vi "AdjustScale.vi"(6 "error in (no error)":errorcluster, 7 "Action":enum16{"Init", "Ignore", "Set Scale"}(ring), 8 "Input Red":dbl, 9 "Red Refnum":refnum<vi>, 10 "Input Blue":dbl, 11 "Blue Refnum":refnum<vi>) -> (4 "error out":errorcluster)   [LabVIEW 2013, in "main.lvlib"]
uses:
  main.lvlib
  <vilib>/Utility/miscctls.llb/LVRangeTypeDef.ctl
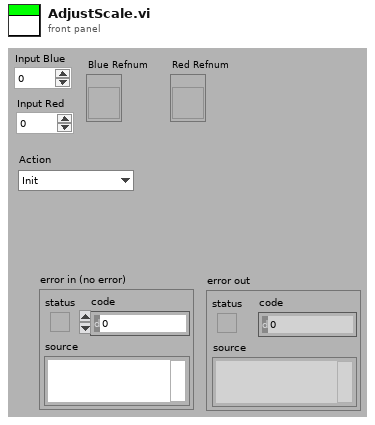
[diagram p1: front panel]
types:
  T1 = typedef "LVRangeTypeDef.ctl" = cluster{"Minimum":dbl, "Maximum":dbl, "Increment":dbl, "Minor Increment":dbl, "Start":dbl}
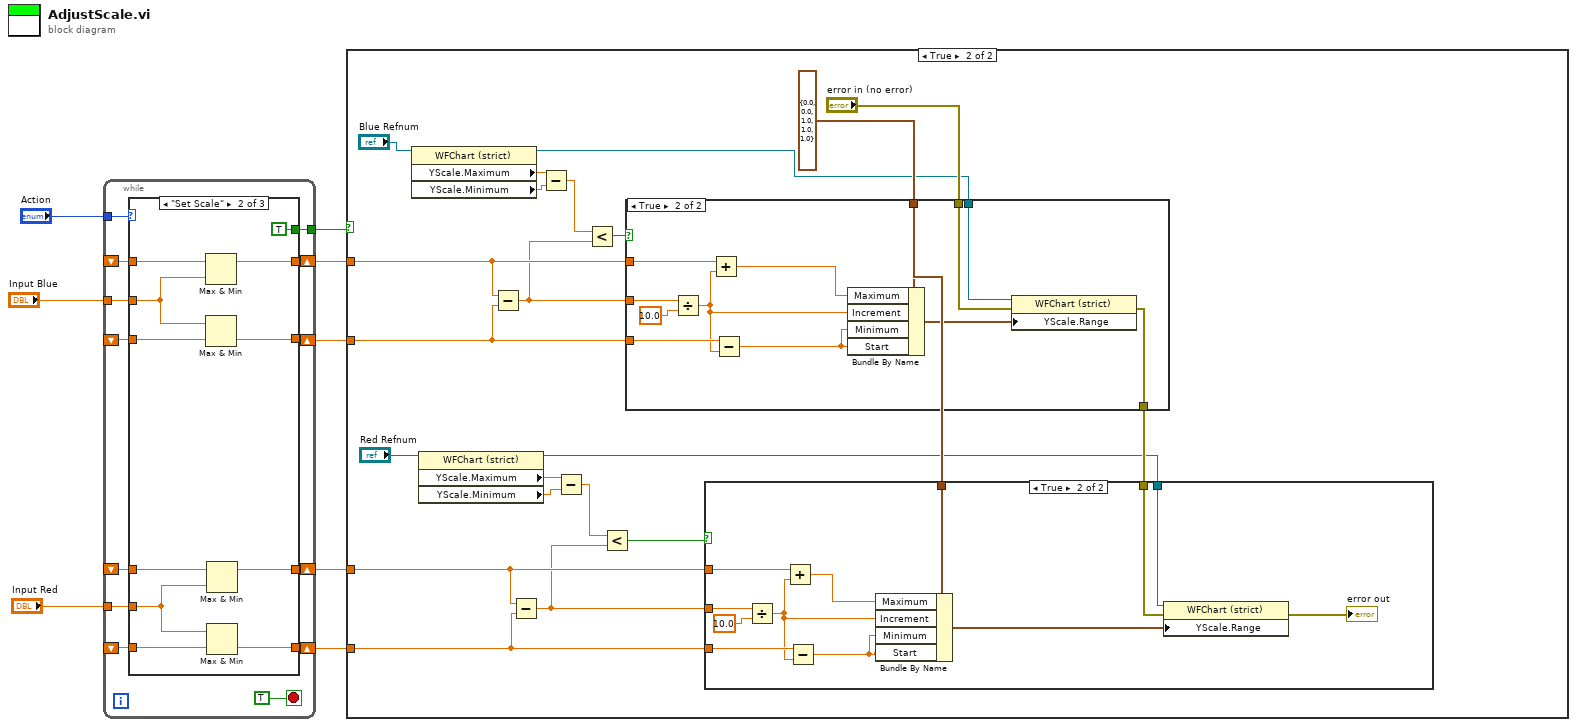
[diagram p0: block diagram]
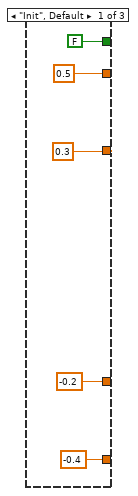
[diagram p5: hidden frame]
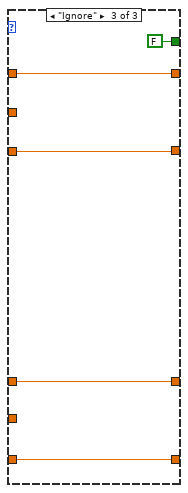
[diagram p6: hidden frame]
diagram:
  n1 = while {
    shift-right: [w19] -> w6
    shift-left: _ -> [w20]
    tunnel: "Input Blue" -> [w21]
    tunnel: "Action" -> [w17]
    shift-right: [w16] -> w5
    shift-left: _ -> [w15]
    shift-right: [w11] -> w3
    shift-left: _ -> [w13]
    shift-right: [w10] -> w2
    shift-left: _ -> [w14]
    tunnel: "Input Red" -> [w12]
    tunnel: [w9] -> w1
    stop <- TRUE stop-if-true
    n2 = case shown="\"Set Scale\"" w17 {
      tunnel: w21 -> [_ w33 _]
      tunnel: w20 -> [_ w37 w41]
      tunnel: [0.5 w36 w41] -> w19
      tunnel: [0.3 w35 w40] -> w16
      tunnel: w15 -> [_ w34 w40]
      tunnel: w14 -> [_ w32 w38]
      tunnel: w13 -> [_ w31 w39]
      tunnel: w12 -> [_ w30 _]
      tunnel: [-0.2 w29 w39] -> w11
      tunnel: [-0.4 w28 w38] -> w10
      tunnel: [FALSE TRUE FALSE] -> w9
      frame "Init", Default {
      }
      frame "Set Scale" {
        n3 = Max & Min(x=w37, y=w33) -> (max(x,y)=w36:dbl)  [unwired: 1 out]
        n4 = Max & Min(x=w33, y=w34) -> (min(x,y)=w35:dbl)  [unwired: 1 out]
        n5 = Max & Min(x=w31, y=w30) -> (max(x,y)=w29:dbl)  [unwired: 1 out]
        n6 = Max & Min(x=w30, y=w32) -> (min(x,y)=w28:dbl)  [unwired: 1 out]
      }
      frame "Ignore" {
      }
    }
  }
  n7 = case shown="True" w1 {
    tunnel: w6 -> [_ w45]
    tunnel: w5 -> [_ w63]
    tunnel: w3 -> [_ w61]
    tunnel: w2 -> [_ w60]
    frame False {
    }
    frame True {
      w62 = T1 {"Minimum"=0.0, "Maximum"=0.0, "Increment"=1.0, "Minor Increment"=1.0, "Start"=1.0} ("Y Scale.Range")
      n8 = property class="WFChart (strict)"(reference="Blue Refnum") -> (reference out=w46:refnum<vi>, "YScale.Maximum"=w50:dbl, "YScale.Minimum"=w49:dbl)  [unwired: 1 in, 1 out]
      n9 = property class="WFChart (strict)"(reference="Red Refnum") -> (reference out=w47:refnum<vi>, "YScale.Maximum"=w55:dbl, "YScale.Minimum"=w56:dbl)  [unwired: 1 in, 1 out]
      n10 = Subtract(x=w45, y=w63) -> (x-y=w44:dbl)
      n11 = Subtract(x=w61, y=w60) -> (x-y=w43:dbl)
      n12 = Subtract(x=w50, y=w49) -> (x-y=w51:dbl)
      n13 = Subtract(x=w55, y=w56) -> (x-y=w54:dbl)
      n14 = Less?(x=w51, y=w44) -> (x < y?=w48:bool)
      n15 = Less?(x=w54, y=w43) -> (x < y?=w53:bool)
      n16 = case shown="True" w48 {
        tunnel: w45 -> [_ w76]
        tunnel: w63 -> [_ w75]
        tunnel: w62 -> [_ w73]
        tunnel: [w64 w71] -> w59
        tunnel: "error in (no error)" -> [w64 w70]
        tunnel: w44 -> [_ w66]
        tunnel: w46 -> [_ w65]
        frame False {
        }
        frame True {
          n17 = Divide(x=w66, y=10.0) -> (x/y=w68:dbl)
          n18 = Add(x=w76, y=w68) -> (x+y=w74:dbl)
          n19 = Subtract(x=w75, y=w68) -> (x-y=w67:dbl)
          n20 = Bundle By Name(cluster=w73, "Maximum"=w74, "Increment"=w68, "Minimum"=w67, "Start"=w67) -> (w72:T1)
          n21 = property class="WFChart (strict)"(reference=w65, error in=w70, "YScale.Range"=w72) -> (error out=w71:errorcluster)  [unwired: 1 out]
        }
      }
      n22 = case shown="True" w53 {
        tunnel: w62 -> [_ w88]
        tunnel: w61 -> [_ w86]
        tunnel: w60 -> [_ w85]
        tunnel: w59 -> [_ w83]
        tunnel: w43 -> [_ w78]
        tunnel: w47 -> [_ w77]
        frame False {
        }
        frame True {
          n23 = Divide(x=w78, y=10.0) -> (x/y=w80:dbl)
          n24 = Add(x=w86, y=w80) -> (x+y=w84:dbl)
          n25 = Subtract(x=w85, y=w80) -> (x-y=w79:dbl)
          n26 = Bundle By Name(cluster=w88, "Maximum"=w84, "Increment"=w80, "Minimum"=w79, "Start"=w79) -> (w87:T1)
          n27 = property class="WFChart (strict)"(reference=w77, error in=w83, "YScale.Range"=w87) -> (error out=→"error out":errorcluster)  [unwired: 1 out]
        }
      }
    }
  }
